vi "Read UART.vi"(7 "UART":u8, 8 "error in (no error)":errorcluster, 9 "Len (LineTerm)":u8, 11 "VISA resource name in":refnum<visa-resource-name>) -> (0 "error out":errorcluster, 1 "Data":string, 3 "VISA resource name":refnum<visa-resource-name>)   [LabVIEW 2024, in "CTIPicoVISA.lvlib"]
uses:
  CTIPicoVISA.lvlib
  <vilib>/Utility/error.llb/Trim Whitespace One-Sided.vi
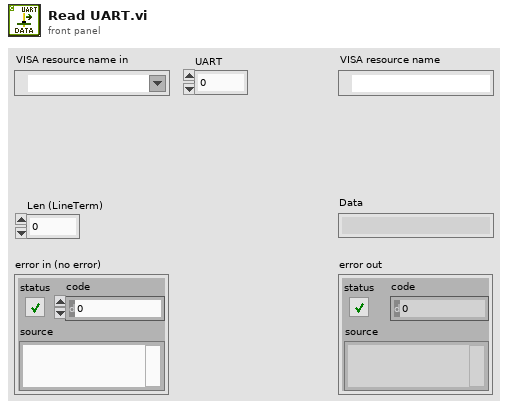
[diagram p1: front panel]
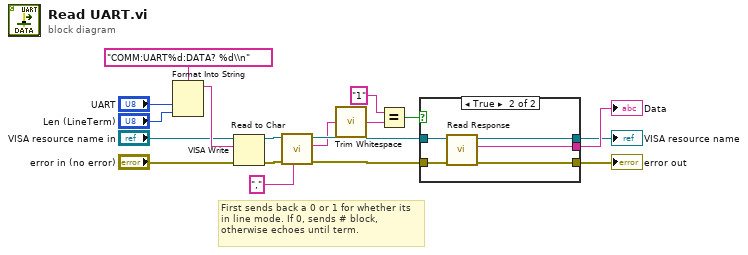
[diagram p0: block diagram]
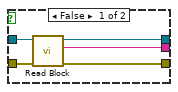
[diagram p2: hidden frame]
diagram:
  # "First sends back a 0 or 1 for whether its in line mode. If 0, sends # block, otherwise echoes until term."
  n1 = Format Into String(format string="COMM:UART%d:DATA? %d\\n", "UART", "Len (LineTerm)") -> (resulting string=w13:string)  [unwired: 2 in, 1 out]
  n2 = VISA Write(VISA resource name="VISA resource name in", write buffer=w13, error in (no error)="error in (no error)") -> (VISA resource name out=w8:refnum<visa-resource-name>, error out=w7:errorcluster)  [unwired: 1 out]
  n3 = call "Read to Char.vi"("Char"=",", "error in (no error)"=w7, "VISA resource name in"=w8) -> ("error out"=w18:errorcluster, "Response"=w2:string, "VISA resource name"=w3:refnum<visa-resource-name>)  [unwired: 6 in]
  n4 = call <vilib>:"Trim Whitespace.vi"("string"=w2) -> ("trimmed string"=w6:string)  [unwired: 1 in]
  n5 = Equal?(x="1" ("y"), y=w6) -> (x = y?=w4:bool)
  n6 = case shown="True" w4 {
    tunnel: [w20 w28] -> w11
    tunnel: [w19 w27] -> w10
    tunnel: [w21 w26] -> w9
    tunnel: w3 -> [w23 w25]
    tunnel: w18 -> [w22 w24]
    frame False {
      n7 = call "Read Block.vi"("error in (no error)"=w22, "VISA resource name in"=w23) -> ("error out"=w21:errorcluster, "Data"=w20:string, "VISA resource name"=w19:refnum<visa-resource-name>)  [unwired: 7 in]
    }
    frame True {
      n8 = call "Read Response.vi"("error in (no error)"=w24, "VISA resource name"=w25) -> ("error out"=w26:errorcluster, "Response"=w28:string, "VISA resource name Out"=w27:refnum<visa-resource-name>)  [unwired: 6 in, 1 out]
    }
  }
  "VISA resource name" <- w10
  "error out" <- w9
  "Data" <- w11
